vi "Get All Monitor DPIs.vi"() -> ()   [LabVIEW 2020, in "MacroAssert.lvlib" / "Win Util.lvlib"]
uses:
  Win Util.lvlib
  MacroAssert.lvlib
panel:
  out "Array":i32[](array[numeric])
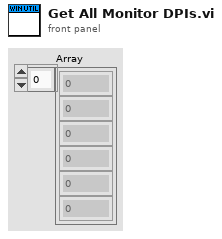
[diagram p1: front panel]
types:
  T1 = cluster{"Left":i32, "Top":i32, "Right":i32, "Bottom":i32}[]
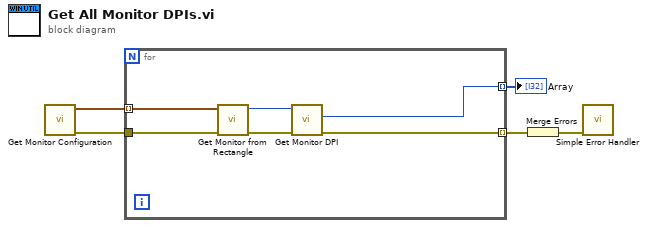
[diagram p0: block diagram]
diagram:
  n1 = call "Get Monitor Configuration.vi"() -> ("error out"=w1:errorcluster, "Display Areas"=w5:T1)  [unwired: 8 in, 2 out]
  n2 = for {
    tunnel: w5 -> [w11] mode=indexing
    tunnel: [w8] -> w4 mode=indexing
    tunnel: [w7] -> w2 mode=indexing
    tunnel: w1 -> [w6]
    n3 = call "Get Monitor from Rectangle.vi"("error in (no error)"=w6, "monitor rect"=w11) -> ("error out"=w10:errorcluster, "HMon"=w9:u32)  [unwired: 8 in]
    n4 = call "Get Monitor DPI.vi"("error in (no error)"=w10, "hMon"=w9) -> ("error out"=w8:errorcluster, "DPI"=w7:i32)  [unwired: 7 in, 1 out]
  }
  "Array" <- w2
  n5 = Merge Errors(w4) -> (w3:errorcluster)
  n6 = call <vilib>:"Simple Error Handler.vi"("error in (no error)"=w3) -> ()  [unwired: 4 in, 5 out]
